vi "Periodic Tasks.vi"(8 "error in 2":errorcluster) -> ()   [LabVIEW 2015]
doc: "This VI runs in parallel to other tasks. It can contain as many user-defined periodic loops as you need. These can carry out PID or other sorts of timed response."
uses:
  <vilib>/Rock Robotics/WPI/Utilities/WPI_GetSetVariantRefNum.vi
panel:
  in  "ARM MAX":dbl
  in  "holdmotor":dbl
  in  "Target Speed (RPM) 2":dbl
  out "Actual Speed (RPM) 2":dbl
  in  "Target Speed (RPM)":dbl
  out "Actual Speed (RPM)":dbl
  in  "target pos":dbl
  out "Actual Pos  2":dbl
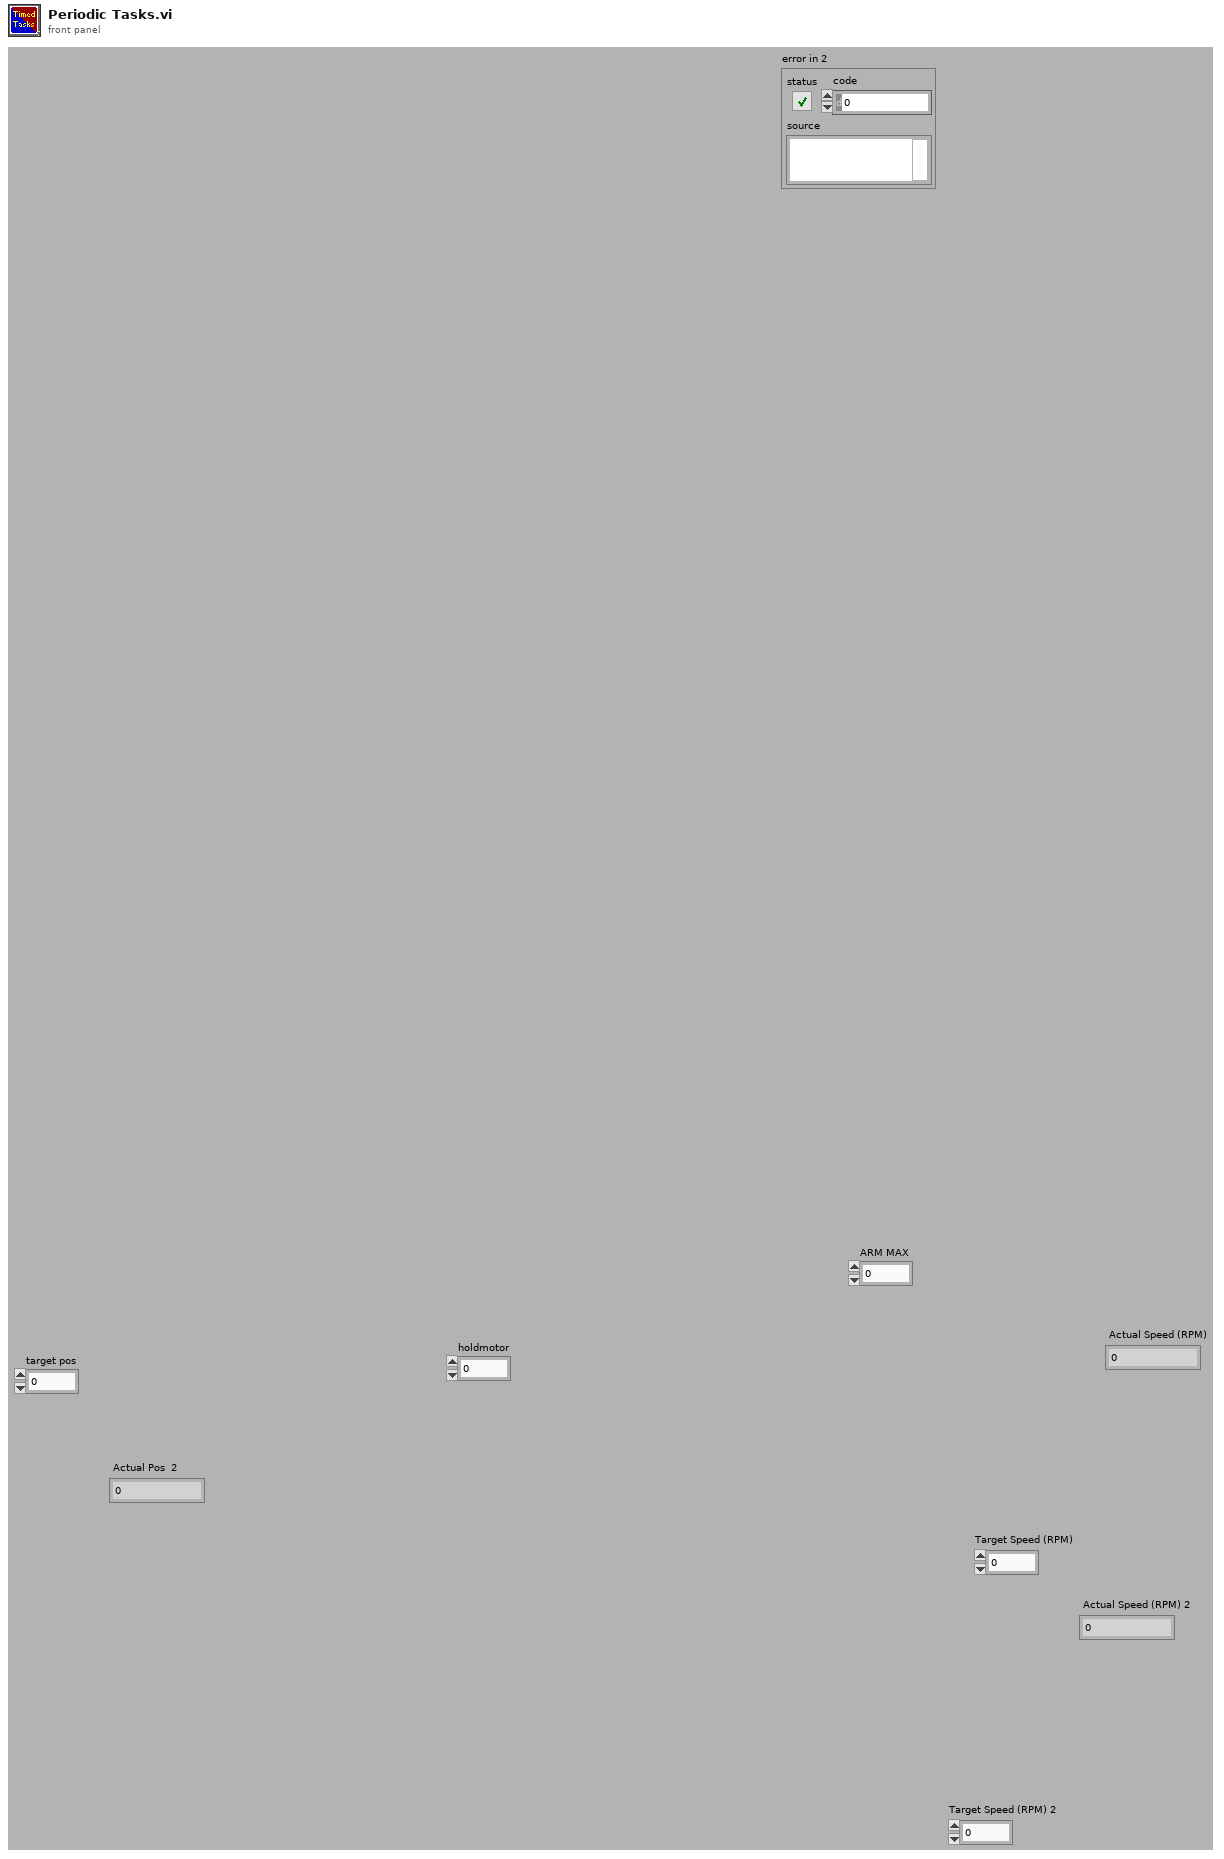
[diagram p1: front panel]
types:
  T1 = typedef "WPI_MotorControlDeviceRef.ctl" = cluster{"DeviceStatus":errorcluster, "Type":T2, "PWM":cluster{"PWM Channel":T3, "DeadBand":T4}, "CAN":cluster{"Device Number":u8, "Control Mode":T5, "Semaphore":T6, "Max Vout":dbl, "TalonSRX Control Mode":T7}, "Invert":bool}
  T2 = typedef "WPI_MotorControlType.ctl" = enum16{"PWM", "CAN", "CANTalonSRX"}
  T3 = typedef "FPGA_DIOPWMChannel.ctl" = enum8{"PWM 0", "PWM 1", "PWM 2", "PWM 3", "PWM 4", "PWM 5", "PWM 6", "PWM 7", "PWM 8", "PWM 9", "PWM MXP 0", "PWM MXP 1", "PWM MXP 2", "PWM MXP 3", "PWM MXP 4", "PWM MXP 5", "PWM MXP 6", "PWM MXP 7", "PWM MXP 8", "PWM MXP 9", "Invalid"}
  T4 = typedef "WPI_PWMDeadband.ctl" = cluster{"Name":string, "maxPositivePwm":i32, "minPositivePwm":i32, "centerPwm":i32, "maxNegativePwm":i32, "minNegativePwm":i32, "angularRange":u16}
  T5 = typedef "WPI_CANJaguar_ControlMode.ctl" = enum8{"Percent VBus", "Current", "Speed", "Position", "Voltage"}
  T6 = typedef "Semaphore RefNum" = refnum<k1>
  T7 = typedef "WPI_CANTalonSRX_APIControlMode.ctl" = enum8{"Percent VBus", "Speed", "Position", "Slave", "Unchanged / Invalid", "Voltage Compensation", "Current", "Motion Profile"}
  T8 = typedef "WPI_SwitchDevRef.ctl" = cluster{"DevStatus":errorcluster, "DIO Channel":T9, "CntIndex":T10, "Normally Closed":bool}
  T9 = typedef "FPGA_DIOChannel.ctl" = enum8{"DIO 0", "DIO 1", "DIO 2", "DIO 3", "DIO 4", "DIO 5", "DIO 6", "DIO 7", "DIO 8", "DIO 9", "DIO MXP 0", "DIO MXP 1", "DIO MXP 2", "DIO MXP 3", "DIO MXP 4", "DIO MXP 5", "DIO MXP 6", "DIO MXP 7", "DIO MXP 8", "DIO MXP 9", "DIO MXP 10", "DIO MXP 11", "DIO MXP 12", "DIO MXP 13", "DIO MXP 14", "DIO MXP 15", "Invalid"}
  T10 = typedef "FPGA_CounterCtrSystemIndex.ctl" = enum8{"Ctr 0", "Ctr 1", "Ctr 2", "Ctr 3", "Ctr 4", "Ctr 5", "Ctr 6", "Ctr 7", "Invalid"}
  T11 = typedef "WPI_JoystickDevRef.ctl" = cluster{"Device":T12}
  T12 = typedef "WPI_JoystickDeviceEnum.ctl" = enum16{"USB 0", "USB 1", "USB 2", "USB 3", "USB 4", "USB 5"}
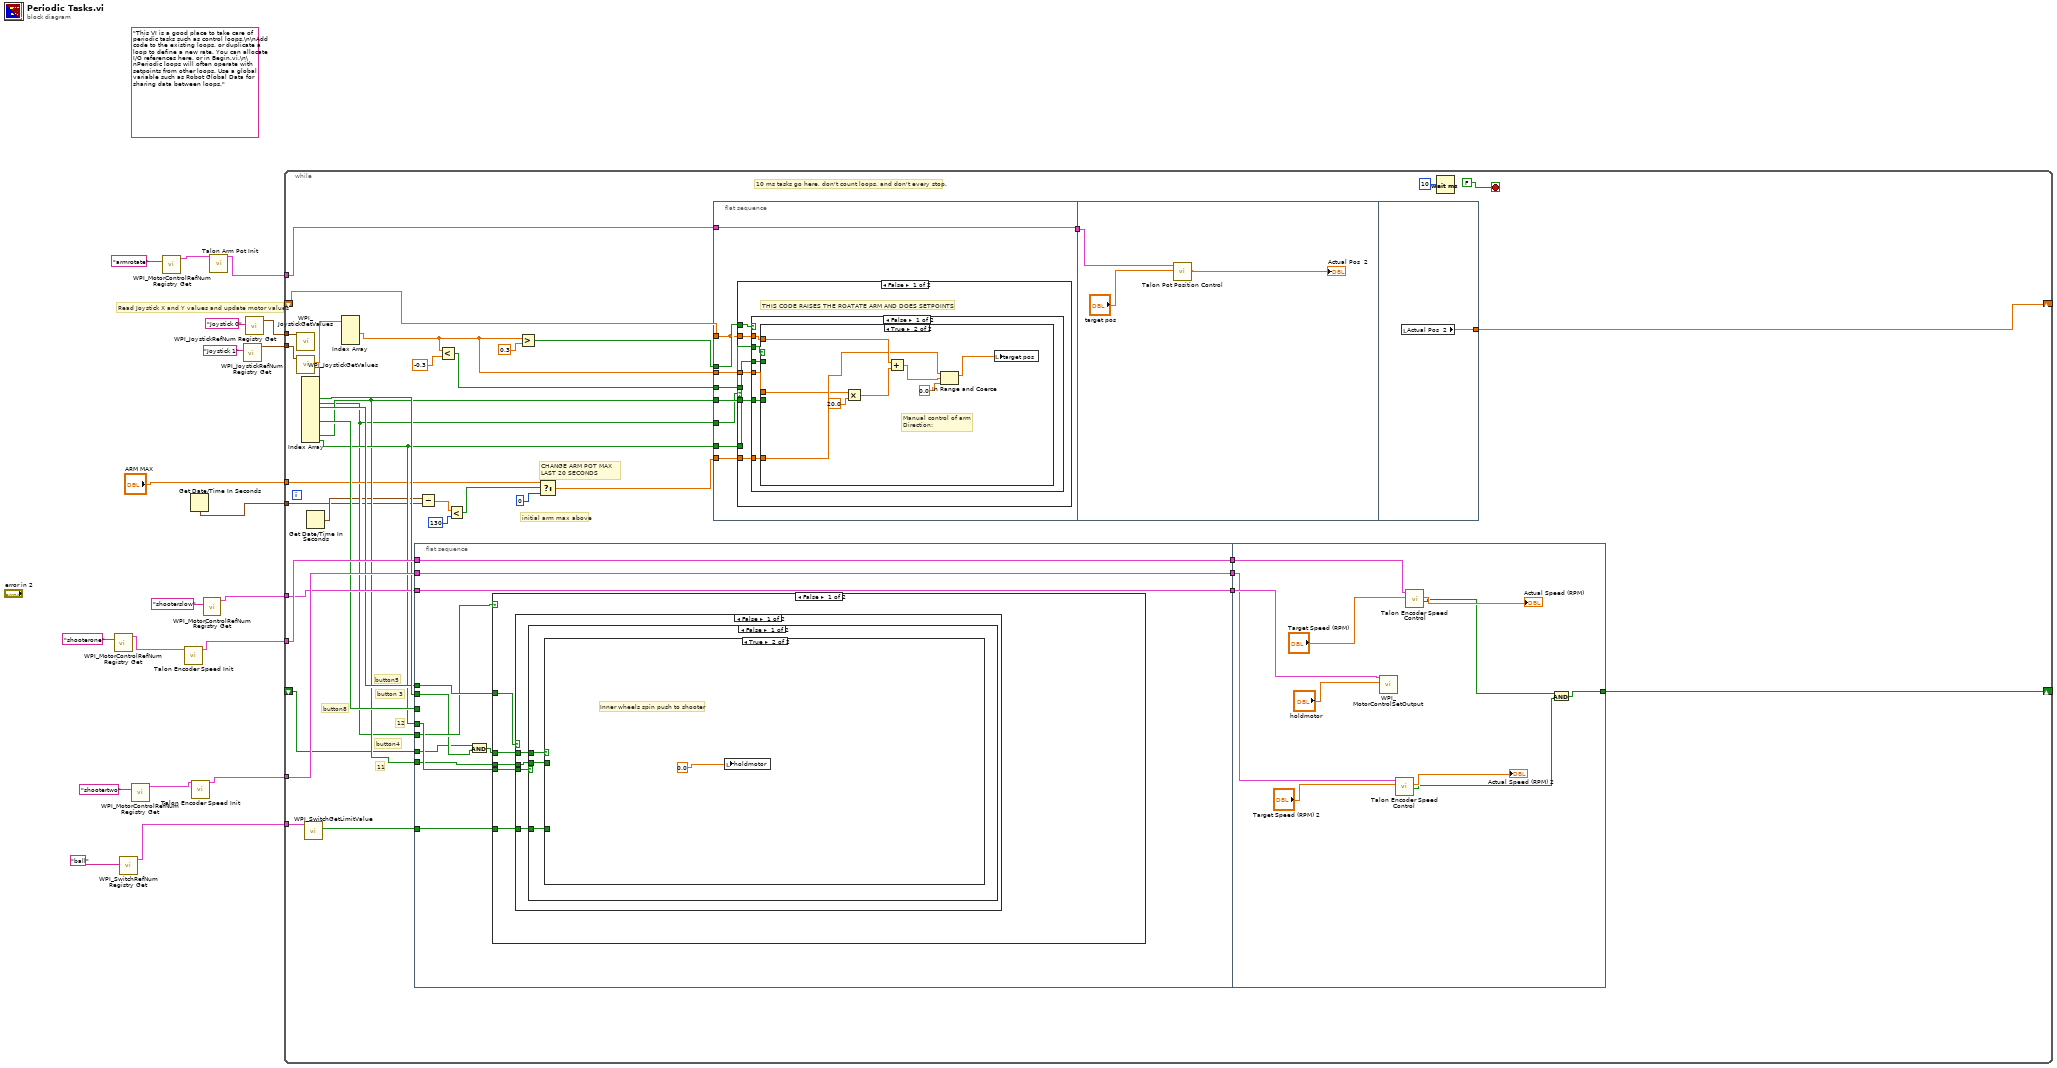
[diagram p0: block diagram]
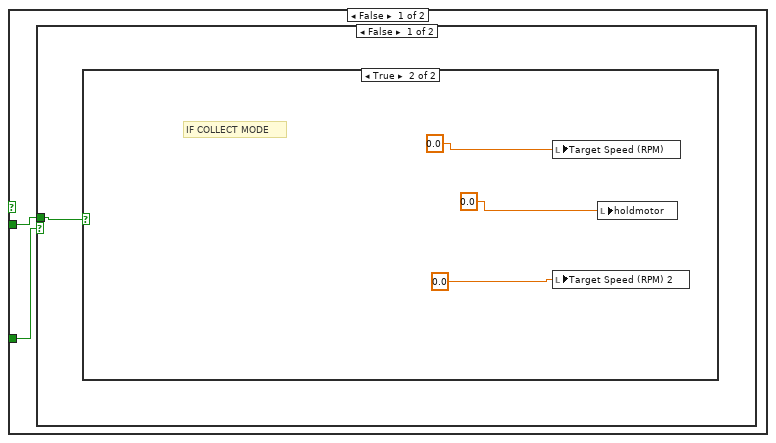
[diagram p2: hidden frame]
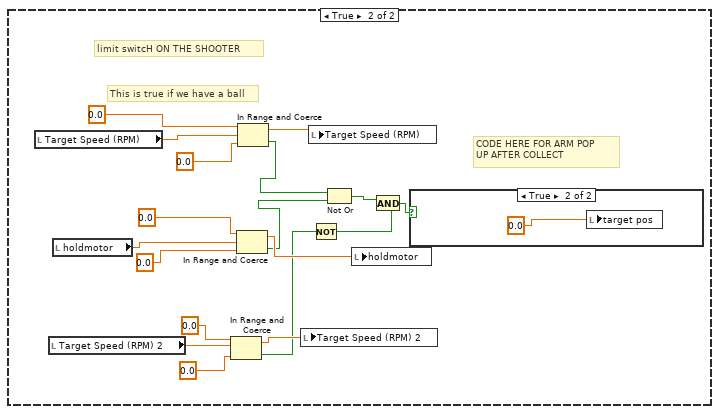
[diagram p4: hidden frame]
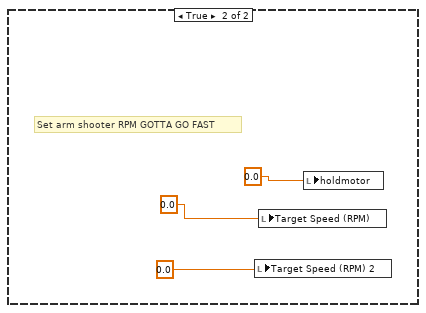
[diagram p6: hidden frame]
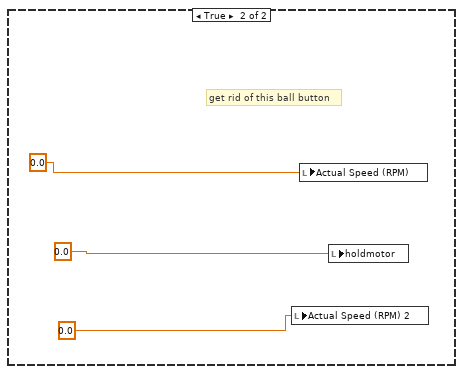
[diagram p7: hidden frame]
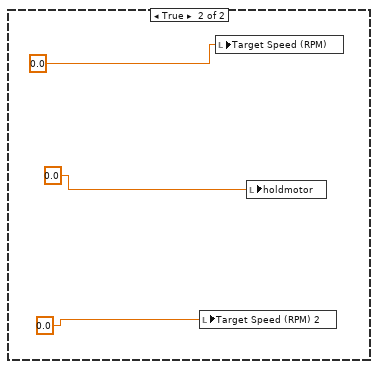
[diagram p8: hidden frame]
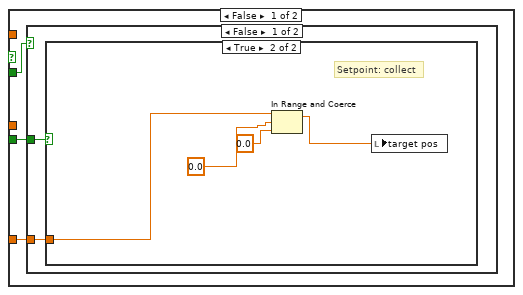
[diagram p9: hidden frame]
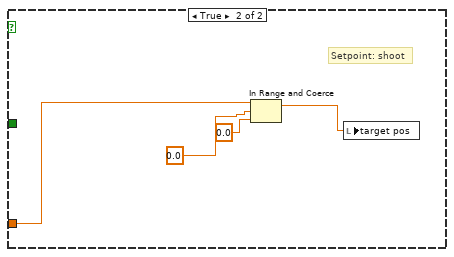
[diagram p11: hidden frame]
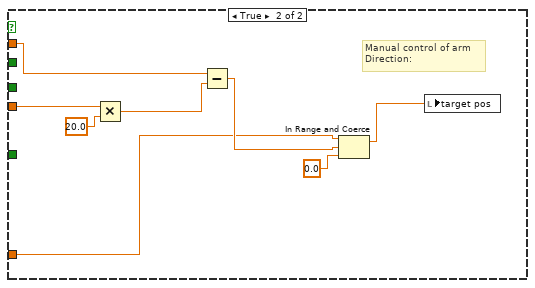
[diagram p12: hidden frame]
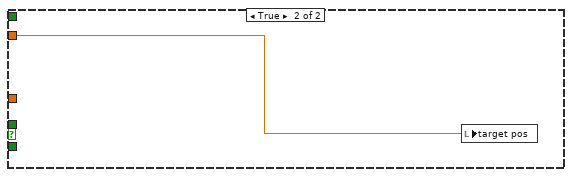
[diagram p13: hidden frame]
diagram:
  (unwired) "This VI is a good place to take care of periodic tasks such as control loops.\n\nAdd code to the existing loops, or duplicate a loop to define a new rate. You can allocate I/O references here, or in Begin.vi.\n\nPeriodic loops will often operate with setpoints from other loops. Use a global variable such as Robot Global Data for sharing data between loops."
  # "Read Joystick X and Y values and update motor values"
  n1 = call <vilib>:"WPI_MotorControlRefNum Registry Get.vi"("refnum name"="shooterone") -> ("MotorControlDevRef"=w7:T1)  [unwired: 9 in, 1 out]
  n2 = call <vilib>:"WPI_SwitchRefNum Registry Get.vi"("refnum name"="ball") -> ("SwitchDevRef"=w3:T8)  [unwired: 9 in, 1 out]
  n3 = call <vilib>:"WPI_MotorControlRefNum Registry Get.vi"("refnum name"="shootertwo") -> ("MotorControlDevRef"=w8:T1)  [unwired: 9 in, 1 out]
  n4 = call <vilib>:"WPI_MotorControlRefNum Registry Get.vi"("refnum name"="armrotate") -> ("MotorControlDevRef"=w5:T1)  [unwired: 9 in, 1 out]
  n5 = call "Talon Encoder Speed Init.vi"("CAN Talon SRX Ref"=w7) -> ("CAN Talon SRX Ref 2"=w6:T1)  [unwired: 9 in, 1 out]
  n6 = Get Date/Time In Seconds() -> (seconds since 1Jan1904=w1:timestamp)
  n7 = call "Talon Encoder Speed Init.vi"("CAN Talon SRX Ref"=w8) -> ("CAN Talon SRX Ref 2"=w9:T1)  [unwired: 9 in, 1 out]
  n8 = call <vilib>:"WPI_MotorControlRefNum Registry Get.vi"("refnum name"="shooterslow") -> ("MotorControlDevRef"=w11:T1)  [unwired: 9 in, 1 out]
  n9 = call "Talon Arm Pot Init.vi"("CAN Talon SRX Ref"=w5) -> ("CAN Talon SRX Ref 2"=w4:T1)  [unwired: 9 in, 1 out]
  n10 = call <vilib>:"WPI_JoystickRefNum Registry Get.vi"("refnum name"="Joystick 1") -> ("JoystickDevRef"=w16:T11)  [unwired: 1 in, 9 out]
  n11 = call <vilib>:"WPI_JoystickRefNum Registry Get.vi"("refnum name"="Joystick 0") -> ("JoystickDevRef"=w18:T11)  [unwired: 1 in, 9 out]
  n12 = while {
    tunnel: w18 -> [w55]
    tunnel: w4 -> [w56]
    tunnel: w16 -> [w54]
    shift-right: [w51] -> _
    shift-left: _ -> [w50]
    tunnel: w9 -> [w48]
    tunnel: w6 -> [w46]
    tunnel: w11 -> [w43]
    tunnel: "ARM MAX" -> [w38]
    tunnel: w3 -> [w36]
    shift-right: [w26] -> _
    shift-left: _ -> [w25]
    tunnel: w1 -> [w21]
    stop <- FALSE stop-if-true
    # "initial arm max above"
    # "CHANGE ARM POT MAX \nLAST 20 SECONDS"
    # "11"
    # "12"
    # "button8"
    # "button4"
    # "button 3"
    # "button5"
    # "10 ms tasks go here, don't count loops, and don't every stop."
    n13 = call <vilib>:"WPI_JoystickGetValues.vi"("JoystickDevRef"=w55) -> ()  [unwired: 6 in, 5 out]
    n14 = call <vilib>:"WPI_JoystickGetValues.vi"("JoystickDevRef"=w54) -> ("Buttons"=w53:bool[], "Axes"=w33:dbl[])  [unwired: 6 in, 3 out]
    n15 = Index Array(array=w53) -> (element #3=w45:bool, element #4=w34:bool, element #5=w42:bool, element #8=w41:bool, element #11=w39:bool, element #12=w40:bool)  [unwired: 12 in, 6 out]
    n16 = call <vilib>:"WPI_SwitchGetLimitValue.vi"("SwitchDevRef"=w36) -> ("Switch Pressed"=w35:bool)  [unwired: 8 in, 2 out]
    n17 = Get Date/Time In Seconds() -> (seconds since 1Jan1904=w22:timestamp)
    n18 = Index Array(array=w33) -> (element #2=w28:dbl)  [unwired: 4 in, 3 out]
    n19 = flat-sequence {
      tunnel: [w69] -> w49
      tunnel: w48 -> [w69]
      tunnel: [w68] -> w47
      tunnel: w46 -> [w68]
      tunnel: w45 -> [w61]
      tunnel: [w67] -> w44
      tunnel: w43 -> [w67]
      tunnel: w42 -> [w66]
      tunnel: w34 -> [w62]
      tunnel: w41 -> [_]
      tunnel: w40 -> [w65]
      tunnel: w39 -> [w63]
      tunnel: w35 -> [w64]
      tunnel: w25 -> [w60]
      tunnel: w49 -> [w122]
      tunnel: w47 -> [w125]
      tunnel: w44 -> [w127]
      tunnel: [w117] -> w26
      frame #0 {
        n20 = And(x=w60, y=w61) -> (x .and. y?=w59:bool)
        n21 = case shown="False" w62 {
          tunnel: w66 -> [w74 _]
          tunnel: w65 -> [w73 _]
          tunnel: w64 -> [w72 _]
          tunnel: w63 -> [w71 _]
          tunnel: w59 -> [w70 _]
          frame False {
            n22 = case shown="False" w74 {
              tunnel: w73 -> [w78 _]
              tunnel: w72 -> [w77 _]
              tunnel: w71 -> [w76 _]
              tunnel: w70 -> [w75 _]
              frame False {
                n23 = case shown="False" w78 {
                  tunnel: w77 -> [w81 _]
                  tunnel: w76 -> [w80 _]
                  tunnel: w75 -> [w79 _]
                  frame False {
                    n24 = case shown="True" w79 {
                      tunnel: w81 -> [w83 _]
                      tunnel: w80 -> [w82 _]
                      frame False {
                        n25 = case shown="False" w83 {
                          tunnel: w82 -> [w84 _]
                          frame False {
                            n26 = case shown="True" w84 {
                              frame False {
                              }
                              frame True {
                                # "IF COLLECT MODE"
                                n27 = local write "Target Speed (RPM)"(0.0) -> ()
                                n28 = local write "Target Speed (RPM) 2"(0.0) -> ()
                                n29 = local write "holdmotor"(0.0) -> ()
                              }
                            }
                          }
                          frame True {
                            # "limit switcH ON THE SHOOTER"
                            # "CODE HERE FOR ARM POP\nUP AFTER COLLECT"
                            # "This is true if we have a ball"
                            n30 = local read "Target Speed (RPM)"() -> (w100:dbl)
                            n31 = local read "Target Speed (RPM) 2"() -> (w98:dbl)
                            n32 = local read "holdmotor"() -> (w99:dbl)
                            n33 = In Range and Coerce(upper limit=0.0, x=w98, lower limit=0.0) -> (coerced(x)=w105:dbl, In Range?=w90:bool)
                            n34 = In Range and Coerce(upper limit=0.0, x=w99, lower limit=0.0) -> (coerced(x)=w104:dbl, In Range?=w92:bool)
                            n35 = In Range and Coerce(upper limit=0.0, x=w100, lower limit=0.0) -> (coerced(x)=w103:dbl, In Range?=w93:bool)
                            n36 = local write "Target Speed (RPM) 2"(w105) -> ()
                            n37 = local write "Target Speed (RPM)"(w103) -> ()
                            n38 = Not(x=w90) -> (.not. x?=w89:bool)
                            n39 = Not Or(1:w92, 2:w93) -> (0:w91:bool)
                            n40 = local write "holdmotor"(w104) -> ()
                            n41 = And(x=w91, y=w89) -> (x .and. y?=w88:bool)
                            n42 = case shown="True" w88 {
                              frame False {
                              }
                              frame True {
                                n43 = local write "target pos"(0.0) -> ()
                              }
                            }
                          }
                        }
                      }
                      frame True {
                        # "Inner wheels spin push to shooter"
                        n44 = local write "holdmotor"(0.0) -> ()
                      }
                    }
                  }
                  frame True {
                    # "Set arm shooter RPM GOTTA GO FAST"
                    n45 = local write "Target Speed (RPM) 2"(0.0) -> ()
                    n46 = local write "Target Speed (RPM)"(0.0) -> ()
                    n47 = local write "holdmotor"(0.0) -> ()
                  }
                }
              }
              frame True {
                # "get rid of this ball button"
                n48 = local write "Actual Speed (RPM) 2"(0.0) -> ()
                n49 = local write "Actual Speed (RPM)"(0.0) -> ()
                n50 = local write "holdmotor"(0.0) -> ()
              }
            }
          }
          frame True {
            n51 = local write "Target Speed (RPM) 2"(0.0) -> ()
            n52 = local write "Target Speed (RPM)"(0.0) -> ()
            n53 = local write "holdmotor"(0.0) -> ()
          }
        }
      }
      frame #1 {
        n54 = call <vilib>:"WPI_MotorControlSetOutput.vi"("Output"="holdmotor", "MotorControlDevRef"=w127) -> ()  [unwired: 7 in, 3 out]
        n55 = call "Talon Encoder Speed Control.vi"("Target Speed (RPM)"="Target Speed (RPM) 2", "MotorControlDevRef"=w122) -> ("Target Speed Reached"=w118:bool, "Actual Speed (RPM)"=→"Actual Speed (RPM) 2":dbl)  [unwired: 6 in, 2 out]
        n56 = call "Talon Encoder Speed Control.vi"("Target Speed (RPM)"="Target Speed (RPM)", "MotorControlDevRef"=w125) -> ("Target Speed Reached"=w119:bool, "Actual Speed (RPM)"=→"Actual Speed (RPM)":dbl)  [unwired: 6 in, 2 out]
        n57 = And(x=w119, y=w118) -> (x .and. y?=w117:bool)
      }
    }
    n58 = Subtract(x=w22, y=w21) -> (x-y=w23:dbl)
    n59 = Less?(x=w28, y=-0.3) -> (x < y?=w29:bool)
    n60 = Less?(x=w23, y=130) -> (x < y?=w24:bool)
    n61 = Greater?(x=w28, y=0.3) -> (0:w31:bool)
    n62 = Select(t=w38, s=w24, f=0) -> (s? t:f=w27:dbl)
    n63 = flat-sequence {
      tunnel: w56 -> [w134]
      tunnel: w31 -> [w136]
      tunnel: w29 -> [w135]
      tunnel: [w134] -> w52
      tunnel: [w133] -> _
      tunnel: w50 -> [w133]
      tunnel: w40 -> [w132]
      tunnel: w39 -> [w131]
      tunnel: w27 -> [w130]
      tunnel: w34 -> [w129]
      tunnel: w28 -> [w128]
      tunnel: w52 -> [w181]
      tunnel: [w183] -> w51
      frame #0 {
        n64 = case shown="False" w129 {
          tunnel: w136 -> [w143 _]
          tunnel: w135 -> [w142 _]
          tunnel: w133 -> [w141 w179]
          tunnel: w132 -> [w140 _]
          tunnel: w131 -> [w139 _]
          tunnel: w130 -> [w138 _]
          tunnel: w128 -> [w137 _]
          frame False {
            # "THIS CODE RAISES THE ROATATE ARM AND DOES SETPOINTS"
            n65 = case shown="False" w143 {
              tunnel: w142 -> [w149 _]
              tunnel: w141 -> [w148 w178]
              tunnel: w140 -> [w147 _]
              tunnel: w139 -> [w146 _]
              tunnel: w138 -> [w145 w174]
              tunnel: w137 -> [w144 w172]
              frame False {
                n66 = case shown="True" w149 {
                  tunnel: w148 -> [_ w170]
                  tunnel: w147 -> [w152 _]
                  tunnel: w146 -> [w151 _]
                  tunnel: w145 -> [w150 w166]
                  tunnel: w144 -> [_ w164]
                  frame False {
                    n67 = case shown="False" w152 {
                      tunnel: w151 -> [w154 _]
                      tunnel: w150 -> [w153 w159]
                      frame False {
                        n68 = case shown="True" w154 {
                          tunnel: w153 -> [_ w155]
                          frame False {
                          }
                          frame True {
                            # "Setpoint: collect"
                            n69 = In Range and Coerce(upper limit=w155, x=0.0, lower limit=0.0) -> (coerced(x)=w156:dbl)  [unwired: 1 out]
                            n70 = local write "target pos"(w156) -> ()
                          }
                        }
                      }
                      frame True {
                        # "Setpoint: shoot"
                        n71 = In Range and Coerce(upper limit=w159, x=0.0, lower limit=0.0) -> (coerced(x)=w160:dbl)  [unwired: 1 out]
                        n72 = local write "target pos"(w160) -> ()
                      }
                    }
                  }
                  frame True {
                    # "Manual control of arm\nDirection:"
                    n73 = Multiply(x=w164, y=20.0) -> (x*y=w163:dbl)
                    n74 = Add(x=w170, y=w163) -> (x+y=w168:dbl)
                    n75 = In Range and Coerce(upper limit=w166, x=w168, lower limit=0.0) -> (coerced(x)=w167:dbl)  [unwired: 1 out]
                    n76 = local write "target pos"(w167) -> ()
                  }
                }
              }
              frame True {
                # "Manual control of arm\nDirection:"
                n77 = Multiply(x=w172, y=20.0) -> (x*y=w171:dbl)
                n78 = Subtract(x=w178, y=w171) -> (x-y=w176:dbl)
                n79 = In Range and Coerce(upper limit=w174, x=w176, lower limit=0.0) -> (coerced(x)=w175:dbl)  [unwired: 1 out]
                n80 = local write "target pos"(w175) -> ()
              }
            }
          }
          frame True {
            n81 = local write "target pos"(w179) -> ()
          }
        }
      }
      frame #1 {
        n82 = call "Talon Pot Position Control.vi"("Target Pos"="target pos", "MotorControlDevRef"=w181) -> ("Actual Pos"=→"Actual Pos  2":dbl)  [unwired: 6 in, 3 out]
      }
      frame #2 {
        n83 = local read "Actual Pos  2"() -> (w183:dbl)
      }
    }
    n84 = Wait (ms)(milliseconds to wait=u32 10) -> ()  [unwired: 1 out]
  }
